vi "Weather Parse Test.vi"() -> ()   [LabVIEW 2020, in "CDM-Config.lvlib"] (continued)
 \"SMALL CRAFT ADVISORY THROUGH WEDNESDAY NIGHT\"\n                    ],\n                    \"BLOCKCHANNEL\": [\n                        \"EAS\",\n                        \"NWEM\",\n                        \"CMAS\"\n                    ],\n                    \"VTEC\": [\n                        \"/O.NEW.PAFC.SC.Y.7456.251203T1400Z-251204T1400Z/\"\n                    ],\n                    \"eventEndingTime\": [\n                        \"2025-12-04T05:00:00-09:00\"\n                    ]\n                },\n                \"scope\": \"Public\",\n                \"code\": \"IPAWSv1.0\",\n                \"language\": \"en-US\",\n                \"web\": \"http://www.weather.gov\",\n                \"eventCode\": {\n                    \"SAME\": [\n                        \"NWS\"\n                    ],\n                    \"NationalWeatherService\": [\n                        \"SCY\"\n                    ]\n                }\n            }\n        },\n        {\n            \"id\": \"https://api.weather.gov/alerts/urn:oid:2.49.0.1.840.0.1f582400c49c338dd966fa4e73bebf0ceb9d5ea9.006.1\",\n            \"type\": \"Feature\",\n            \"geometry\": null,\n            \"properties\": {\n                \"@id\": \"https://api.weather.gov/alerts/urn:oid:2.49.0.1.840.0.1f582400c49c338dd966fa4e73bebf0ceb9d5ea9.006.1\",\n                \"@type\": \"wx:Alert\",\n                \"id\": \"urn:oid:2.49.0.1.840.0.1f582400c49c338dd966fa4e73bebf0ceb9d5ea9.006.1\",\n                \"areaDesc\": \"Cape Cleare to Gore Point from 15 to 75 NM\",\n                \"geocode\": {\n                    \"SAME\": [\n                        \"058716\"\n                    ],\n                    \"UGC\": [\n                        \"PKZ716\"\n                    ]\n                },\n                \"affectedZones\": [\n                    \"https://api.weather.gov/zones/forecast/PKZ716\"\n                ],\n                \"references\": [],\n                \"sent\": \"2025-12-02T15:47:00-09:00\",\n                \"effective\": \"2025-12-02T15:47:00-09:00\",\n                \"onset\": \"2025-12-03T05:00:00-09:00\",\n                \"expires\": \"2025-12-03T04:45:00-09:00\",\n                \"ends\": \"2025-12-04T05:00:00-09:00\",\n                \"status\": \"Actual\",\n                \"messageType\": \"Alert\",\n                \"category\": \"Met\",\n                \"severity\": \"Minor\",\n                \"certainty\": \"Likely\",\n                \"urgency\": \"Expected\",\n                \"event\": \"Small Craft Advisory\",\n                \"sender\": \"w-nws.webmaster@noaa.gov\",\n                \"senderName\": \"NWS Anchorage AK\",\n                \"headline\": \"Small Craft Advisory issued December 2 at 3:47PM AKST until December 4 at 5:00AM AKST by NWS Anchorage AK\",\n                \"description\": \"Coastal Waters Forecast for the Northern Gulf of Alaska Coast\\nup to 100 nm out including Kodiak Island and Cook Inlet.\\n\\nWind forecasts reflect the predominant speed and direction\\nexpected. Sea forecasts represent an average of the highest\\none-third of the combined wind wave and swell height.\\n\\n.TONIGHT...Variable wind 10 kt. Seas 11 ft.\\n.WED...Variable wind 10 kt. Seas 10 ft.\\n.WED NIGHT...SW wind 15 kt. Seas 10 ft.\\n.THU AND THU NIGHT...Variable wind 10 kt. Seas 8 ft.\\n.FRI...NW wind 20 kt. Seas 6 ft.\\n.SAT...SE wind 15 kt. Seas 7 ft.\\n.SUN...E wind 15 kt. Seas 11 ft.\",\n                \"instruction\": null,\n                \"response\": \"Avoid\",\n                \"parameters\": {\n                    \"AWIPSidentifier\": [\n                        \"CWFAER\"\n                    ],\n                    \"WMOidentifier\": [\n                        \"FZAK51 PAFC 030047\"\n                    ],\n                    \"NWSheadline\": [\n                        \"SMALL CRAFT ADVISORY THROUGH WEDNESDAY NIGHT\"\n                    ],\n                    \"BLOCKCHANNEL\": [\n                        \"EAS\",\n                        \"NWEM\",\n                        \"CMAS\"\n                    ],\n                    \"VTEC\": [\n                        \"/O.NEW.PAFC.SC.Y.7452.251203T1400Z-251204T1400Z/\"\n                    ],\n                    \"eventEndingTime\": [\n                        \"2025-12-04T05:00:00-09:00\"\n                    ]\n                },\n                \"scope\": \"Public\",\n                \"code\": \"IPAWSv1.0\",\n                \"language\": \"en-US\",\n                \"web\": \"http://www.weather.gov\",\n                \"eventCode\": {\n                    \"SAME\": [\n                        \"NWS\"\n                    ],\n                    \"NationalWeatherService\": [\n                        \"SCY\"\n                    ]\n                }\n            }\n        },\n        {\n            \"id\": \"https://api.weather.gov/alerts/urn:oid:2.49.0.1.840.0.1f582400c49c338dd966fa4e73bebf0ceb9d5ea9.017.1\",\n            \"type\": \"Feature\",\n            \"geometry\": null,\n            \"properties\": {\n                \"@id\": \"https://api.weather.gov/alerts/urn:oid:2.49.0.1.840.0.1f582400c49c338dd966fa4e73bebf0ceb9d5ea9.017.1\",\n                \"@type\": \"wx:Alert\",\n                \"id\": \"urn:oid:2.49.0.1.840.0.1f582400c49c338dd966fa4e73bebf0ceb9d5ea9.017.1\",\n                \"areaDesc\": \"Gore Point to Marmot Island from 15 to 80 NM\",\n                \"geocode\": {\n                    \"SAME\": [\n                        \"058733\"\n                    ],\n                    \"UGC\": [\n                        \"PKZ733\"\n                    ]\n                },\n                \"affectedZones\": [\n                    \"https://api.weather.gov/zones/forecast/PKZ733\"\n                ],\n                \"references\": [],\n                \"sent\": \"2025-12-02T15:47:00-09:00\",\n                \"effective\": \"2025-12-02T15:47:00-09:00\",\n                \"onset\": \"2025-12-03T05:00:00-09:00\",\n                \"expires\": \"2025-12-03T04:45:00-09:00\",\n                \"ends\": \"2025-12-04T05:00:00-09:00\",\n                \"status\": \"Actual\",\n                \"messageType\": \"Alert\",\n                \"category\": \"Met\",\n                \"severity\": \"Minor\",\n                \"certainty\": \"Likely\",\n                \"urgency\": \"Expected\",\n                \"event\": \"Small Craft Advisory\",\n                \"sender\": \"w-nws.webmaster@noaa.gov\",\n                \"senderName\": \"NWS Anchorage AK\",\n                \"headline\": \"Small Craft Advisory issued December 2 at 3:47PM AKST until December 4 at 5:00AM AKST by NWS Anchorage AK\",\n                \"description\": \"Coastal Waters Forecast for the Northern Gulf of Alaska Coast\\nup to 100 nm out including Kodiak Island and Cook Inlet.\\n\\nWind forecasts reflect the predominant speed and direction\\nexpected. Sea forecasts represent an average of the highest\\none-third of the combined wind wave and swell height.\\n\\n.TONIGHT...SE wind 15 kt. Seas 11 ft.\\n.WED...SE wind 15 kt. Seas 11 ft.\\n.WED NIGHT...SW wind 15 kt. Seas 9 ft.\\n.THU...SW wind 15 kt. Seas 8 ft.\\n.THU NIGHT...Variable wind 10 kt. Seas 7 ft.\\n.FRI...NW wind 15 kt. Seas 9 ft.\\n.SAT...Variable wind 10 kt. Seas 9 ft.\\n.SUN...E wind 15 kt. Seas 9 ft.\",\n                \"instruction\": null,\n                \"response\": \"Avoid\",\n                \"parameters\": {\n                    \"AWIPSidentifier\": [\n                        \"CWFAER\"\n                    ],\n                    \"WMOidentifier\": [\n                        \"FZAK51 PAFC 030047\"\n                    ],\n                    \"NWSheadline\": [\n                        \"SMALL CRAFT ADVISORY THROUGH WEDNESDAY NIGHT\"\n                    ],\n                    \"BLOCKCHANNEL\": [\n                        \"EAS\",\n                        \"NWEM\",\n                        \"CMAS\"\n                    ],\n                    \"VTEC\": [\n                        \"/O.NEW.PAFC.SC.Y.7454.251203T1400Z-251204T1400Z/\"\n                    ],\n                    \"eventEndingTime\": [\n                        \"2025-12-04T05:00:00-09:00\"\n                    ]\n                },\n                \"scope\": \"Public\",\n                \"code\": \"IPAWSv1.0\",\n                \"language\": \"en-US\",\n                \"web\": \"http://www.weather.gov\",\n                \"eventCode\": {\n                    \"SAME\": [\n                        \"NWS\"\n                    ],\n                    \"NationalWeatherService\": [\n                        \"SCY\"\n                    ]\n                }\n            }\n        },\n        {\n            \"id\": \"https://api.weather.gov/alerts/urn:oid:2.49.0.1.840.0.1f582400c49c338dd966fa4e73bebf0ceb9d5ea9.003.1\",\n            \"type\": \"Feature\",\n            \"geometry\": null,\n            \"properties\": {\n                \"@id\": \"https://api.weather.gov/alerts/urn:oid:2.49.0.1.840.0.1f582400c49c338dd966fa4e73bebf0ceb9d5ea9.003.1\",\n                \"@type\": \"wx:Alert\",\n                \"id\": \"urn:oid:2.49.0.1.840.0.1f582400c49c338dd966fa4e73bebf0ceb9d5ea9.003.1\",\n                \"areaDesc\": \"Gravel Point to Cape Cleare out to 15 NM\",\n                \"geocode\": {\n                    \"SAME\": [\n                        \"058711\"\n                    ],\n                    \"UGC\": [\n                        \"PKZ711\"\n                    ]\n                },\n                \"affectedZones\": [\n                    \"https://api.weather.gov/zones/forecast/PKZ711\"\n                ],\n                \"references\": [],\n                \"sent\": \"2025-12-02T15:47:00-09:00\",\n                \"effective\": \"2025-12-02T15:47:00-09:00\",\n                \"onset\": \"2025-12-03T05:00:00-09:00\",\n                \"expires\": \"2025-12-03T04:45:00-09:00\",\n                \"ends\": \"2025-12-04T05:00:00-09:00\",\n                \"status\": \"Actual\",\n                \"messageType\": \"Alert\",\n                \"category\": \"Met\",\n                \"severity\": \"Minor\",\n                \"certainty\": \"Likely\",\n                \"urgency\": \"Expected\",\n                \"event\": \"Small Craft Advisory\",\n                \"sender\": \"w-nws.webmaster@noaa.gov\",\n                \"senderName\": \"NWS Anchorage AK\",\n                \"headline\": \"Small Craft Advisory issued December 2 at 3:47PM AKST until December 4 at 5:00AM AKST by NWS Anchorage AK\",\n                \"description\": \"Coastal Waters Forecast for the Northern Gulf of Alaska Coast\\nup to 100 nm out including Kodiak Island and Cook Inlet.\\n\\nWind forecasts reflect the predominant speed and direction\\nexpected. Sea forecasts represent an average of the highest\\none-third of the combined wind wave and swell height.\\n\\n.TONIGHT...SE wind 25 kt. Seas 10 ft.\\n.WED...SE wind 15 kt in the morning becoming variable 10 kt. Seas\\n10 ft. Rain.\\n.WED NIGHT...Variable wind 10 kt. Seas 9 ft.\\n.THU...Variable wind 10 kt. Seas 7 ft.\\n.THU NIGHT...Variable wind 10 kt. Seas 6 ft.\\n.FRI...NE wind 15 kt. Seas 6 ft.\\n.SAT THROUGH SUN...E wind 20 kt. Seas 10 ft.\",\n                \"instruction\": null,\n                \"response\": \"Avoid\",\n                \"parameters\": {\n                    \"AWIPSidentifier\": [\n                        \"CWFAER\"\n                    ],\n                    \"WMOidentifier\": [\n                        \"FZAK51 PAFC 030047\"\n                    ],\n                    \"NWSheadline\": [\n                        \"SMALL CRAFT ADVISORY THROUGH WEDNESDAY NIGHT\"\n                    ],\n                    \"BLOCKCHANNEL\": [\n                        \"EAS\",\n                        \"NWEM\",\n                        \"CMAS\"\n                    ],\n                    \"VTEC\": [\n                        \"/O.NEW.PAFC.SC.Y.7449.251203T1400Z-251204T1400Z/\"\n                    ],\n                    \"eventEndingTime\": [\n                        \"2025-12-04T05:00:00-09:00\"\n                    ]\n                },\n                \"scope\": \"Public\",\n                \"code\": \"IPAWSv1.0\",\n                \"language\": \"en-US\",\n                \"web\": \"http://www.weather.gov\",\n                \"eventCode\": {\n                    \"SAME\": [\n                        \"NWS\"\n                    ],\n                    \"NationalWeatherService\": [\n                        \"SCY\"\n                    ]\n                }\n            }\n        },\n        {\n            \"id\": \"https://api.weather.gov/alerts/urn:oid:2.49.0.1.840.0.1f582400c49c338dd966fa4e73bebf0ceb9d5ea9.018.1\",\n            \"type\": \"Feature\",\n            \"geometry\": null,\n            \"properties\": {\n                \"@id\": \"https://api.weather.gov/alerts/urn:oid:2.49.0.1.840.0.1f582400c49c338dd966fa4e73bebf0ceb9d5ea9.018.1\",\n                \"@type\": \"wx:Alert\",\n                \"id\": \"urn:oid:2.49.0.1.840.0.1f582400c49c338dd966fa4e73bebf0ceb9d5ea9.018.1\",\n                \"areaDesc\": \"Marmot Island to Sitkinak out to 15 NM\",\n                \"geocode\": {\n                    \"SAME\": [\n                        \"058732\"\n                    ],\n                    \"UGC\": [\n                        \"PKZ732\"\n                    ]\n                },\n                \"affectedZones\": [\n                    \"https://api.weather.gov/zones/forecast/PKZ732\"\n                ],\n                \"references\": [],\n                \"sent\": \"2025-12-02T15:47:00-09:00\",\n                \"effective\": \"2025-12-02T15:47:00-09:00\",\n                \"onset\": \"2025-12-03T05:00:00-09:00\",\n                \"expires\": \"2025-12-03T04:45:00-09:00\",\n                \"ends\": \"2025-12-04T05:00:00-09:00\",\n                \"status\": \"Actual\",\n                \"messageType\": \"Alert\",\n                \"category\": \"Met\",\n                \"severity\": \"Minor\",\n                \"certainty\": \"Likely\",\n                \"urgency\": \"Expected\",\n                \"event\": \"Small Craft Advisory\",\n                \"sender\": \"w-nws.webmaster@noaa.gov\",\n                \"senderName\": \"NWS Anchorage AK\",\n                \"headline\": \"Small Craft Advisory issued December 2 at 3:47PM AKST until December 4 at 5:00AM AKST by NWS Anchorage AK\",\n                \"description\": \"Coastal Waters Forecast for the Northern Gulf of Alaska Coast\\nup to 100 nm out including Kodiak Island and Cook Inlet.\\n\\nWind forecasts reflect the predominant speed and direction\\nexpected. Sea forecasts represent an average of the highest\\none-third of the combined wind wave and swell height.\\n\\n.TONIGHT...E wind 20 kt. Seas 13 ft.\\n.WED...S wind 20 kt. Seas 12 ft.\\n.WED NIGHT...S wind 15 kt. Seas 9 ft.\\n.THU...SE wind 15 kt. Seas 9 ft.\\n.THU NIGHT...NE wind 20 kt. Seas 9 ft.\\n.FRI THROUGH SUN...W wind 20 kt. Seas 7 ft.\",\n                \"instruction\": null,\n                \"response\": \"Avoid\",\n                \"parameters\": {\n                    \"AWIPSidentifier\": [\n                        \"CWFAER\"\n                    ],\n                    \"WMOidentifier\": [\n                        \"FZAK51 PAFC 030047\"\n                    ],\n                    \"NWSheadline\": [\n                        \"SMALL CRAFT ADVISORY THROUGH WEDNESDAY NIGHT\"\n                    ],\n                    \"BLOCKCHANNEL\": [\n                        \"EAS\",\n                        \"NWEM\",\n                        \"CMAS\"\n                    ],\n                    \"VTEC\": [\n                        \"/O.NEW.PAFC.SC.Y.7455.251203T1400Z-251204T1400Z/\"\n                    ],\n                    \"eventEndingTime\": [\n                        \"2025-12-04T05:00:00-09:00\"\n                    ]\n                },\n                \"scope\": \"Public\",\n                \"code\": \"IPAWSv1.0\",\n                \"language\": \"en-US\",\n                \"web\": \"http://www.weather.gov\",\n                \"eventCode\": {\n                    \"SAME\": [\n                        \"NWS\"\n                    ],\n                    \"NationalWeatherService\": [\n                        \"SCY\"\n                    ]\n                }\n            }\n        },\n        {\n            \"id\": \"https://api.weather.gov/alerts/urn:oid:2.49.0.1.840.0.1f582400c49c338dd966fa4e73bebf0ceb9d5ea9.004.1\",\n            \"type\": \"Feature\",\n            \"geometry\": null,\n            \"properties\": {\n                \"@id\": \"https://api.weather.gov/alerts/urn:oid:2.49.0.1.840.0.1f582400c49c338dd966fa4e73bebf0ceb9d5ea9.004.1\",\n                \"@type\": \"wx:Alert\",\n                \"id\": \"urn:oid:2.49.0.1.840.0.1f582400c49c338dd966fa4e73bebf0ceb9d5ea9.004.1\",\n                \"areaDesc\": \"Cape Suckling to Cape Cleare from 15 to 75 NM\",\n                \"geocode\": {\n                    \"SAME\": [\n                        \"058712\"\n                    ],\n                    \"UGC\": [\n                        \"PKZ712\"\n                    ]\n                },\n                \"affectedZones\": [\n                    \"https://api.weather.gov/zones/forecast/PKZ712\"\n                ],\n                \"references\": [],\n                \"sent\": \"2025-12-02T15:47:00-09:00\",\n                \"effective\": \"2025-12-02T15:47:00-09:00\",\n                \"onset\": \"2025-12-03T05:00:00-09:00\",\n                \"expires\": \"2025-12-03T04:45:00-09:00\",\n                \"ends\": \"2025-12-04T05:00:00-09:00\",\n                \"status\": \"Actual\",\n                \"messageType\": \"Alert\",\n                \"category\": \"Met\",\n                \"severity\": \"Minor\",\n                \"certainty\": \"Likely\",\n                \"urgency\": \"Expected\",\n                \"event\": \"Small Craft Advisory\",\n                \"sender\": \"w-nws.webmaster@noaa.gov\",\n                \"senderName\": \"NWS Anchorage AK\",\n                \"headline\": \"Small Craft Advisory issued December 2 at 3:47PM AKST until December 4 at 5:00AM AKST by NWS Anchorage AK\",\n                \"description\": \"Coastal Waters Forecast for the Northern Gulf of Alaska Coast\\nup to 100 nm out including Kodiak Island and Cook Inlet.\\n\\nWind forecasts reflect the predominant speed and direction\\nexpected. Sea forecasts represent an average of the highest\\none-third of the combined wind wave and swell height.\\n\\n.TONIGHT...SE wind 25 kt. Seas 10 ft.\\n.WED...S wind 15 kt. Seas 11 ft.\\n.WED NIGHT...SW wind 15 kt. Seas 10 ft.\\n.THU...SW wind 15 kt. Seas 8 ft.\\n.THU NIGHT...Variable wind 10 kt. Seas 8 ft.\\n.FRI...S wind 15 kt. Seas 7 ft.\\n.SAT THROUGH SUN...SE wind 20 kt. Seas 11 ft.\",\n                \"instruction\": null,\n                \"response\": \"Avoid\",\n                \"parameters\": {\n                    \"AWIPSidentifier\": [\n                        \"CWFAER\"\n                    ],\n                    \"WMOidentifier\": [\n                        \"FZAK51 PAFC 030047\"\n                    ],\n                    \"NWSheadline\": [\n                        \"SMALL CRAFT ADVISORY THROUGH WEDNESDAY NIGHT\"\n                    ],\n                    \"BLOCKCHANNEL\": [\n                        \"EAS\",\n                        \"NWEM\",\n                        \"CMAS\"\n                    ],\n                    \"VTEC\": [\n                        \"/O.NEW.PAFC.SC.Y.7450.251203T1400Z-251204T1400Z/\"\n                    ],\n                    \"eventEndingTime\": [\n                        \"2025-12-04T05:00:00-09:00\"\n                    ]\n                },\n                \"scope\": \"Public\",\n                \"code\": \"IPAWSv1.0\",\n                \"language\": \"en-US\",\n                \"web\": \"http://www.weather.gov\",\n                \"eventCode\": {\n                    \"SAME\": [\n                        \"NWS\"\n                    ],\n                    \"NationalWeatherService\": [\n                        \"SCY\"\n                    ]\n                }\n            }\n        },\n        {\n            \"id\": \"https://api.weather.gov/alerts/urn:oid:2.49.0.1.840.0.ddc072ff7c65d7dc76b55ecdda687f2ed71d6895.001.1\",\n            \"type\": \"Feature\",\n            \"geometry\": null,\n            \"properties\": {\n                \"@id\": \"https://api.weather.gov/alerts/urn:oid:2.49.0.1.840.0.ddc072ff7c65d7dc76b55ecdda687f2ed71d6895.001.1\",\n                \"@type\": \"wx:Alert\",\n                \"id\": \"urn:oid:2.49.0.1.840.0.ddc072ff7c65d7dc76b55ecdda687f2ed71d6895.001.1\",\n                \"areaDesc\": \"Yakutat Bay\",\n                \"geocode\": {\n                    \"SAME\": [\n                        \"058053\"\n                    ],\n                    \"UGC\": [\n                        \"PKZ053\"\n                    ]\n                },\n                \"affectedZones\": [\n                    \"https://api.weather.gov/zones/forecast/PKZ053\"\n                ],\n                \"references\": [],\n                \"sent\": \"2025-12-02T14:58:00-09:00\",\n                \"effective\": \"2025-12-02T14:58:00-09:00\",\n                \"onset\": \"2025-12-02T14:00:00-09:00\",\n                \"expires\": \"2025-12-03T09:00:00-09:00\",\n                \"ends\": \"2025-12-03T17:00:00-09:00\",\n                \"status\": \"Actual\",\n                \"messageType\": \"Alert\",\n                \"category\": \"Met\",\n                \"severity\": \"Minor\",\n                \"certainty\": \"Likely\",\n                \"urgency\": \"Expected\",\n                \"event\": \"Small Craft Advisory\",\n                \"sender\": \"w-nws.webmaster@noaa.gov\",\n                \"senderName\": \"NWS Juneau AK\",\n                \"headline\": \"Small Craft Advisory issued December 2 at 2:58PM AKST until December 3 at 5:00PM AKST by NWS Juneau AK\",\n                \"description\": \"Coastal Waters Forecast for Yakutat Bay\\n\\nWind forecasts reflect the predominant speed and direction\\nexpected. Sea forecasts represent the average of the highest\\none-third of the combined windwave and swell height.\\n\\n.TONIGHT...E wind 15 kt. Seas 9 ft. Rain.\\n.WED...E wind 15 kt. Seas 10 ft. S swell. Rain.\\n.WED NIGHT...S wind 10 kt in the evening becoming light.\\nSeas 9 ft. S swell. Rain.\\n.THU...E wind 10 kt. Seas 8 ft. SW swell. Rain.\\n.THU NIGHT...E wind 15 kt. Seas 7 ft. SW swell. Rain.\\n.FRI...E wind 25 kt. Seas 7 ft.\\n.SAT...E gale to 35 kt. Seas 10 ft.\\n.SUN...E gale to 35 kt. Seas 12 ft.\",\n                \"instruction\": null,\n                \"response\": \"Avoid\",\n                \"parameters\": {\n                    \"AWIPSidentifier\": [\n                        \"CWFYAK\"\n                    ],\n                    \"WMOidentifier\": [\n                        \"FZAK53 PAJK 022358\"\n                    ],\n                    \"NWSheadline\": [\n                        \"SMALL CRAFT ADVISORY THROUGH WEDNESDAY\"\n                    ],\n                    \"BLOCKCHANNEL\": [\n                        \"EAS\",\n                        \"NWEM\",\n                        \"CMAS\"\n                    ],\n                    \"VTEC\": [\n                        \"/O.NEW.PAJK.SC.Y.5129.251202T2300Z-251204T0200Z/\"\n                    ],\n                    \"eventEndingTime\": [\n                        \"2025-12-03T17:00:00-09:00\"\n                    ]\n                },\n                \"scope\": \"Public\",\n                \"code\": \"IPAWSv1.0\",\n                \"language\": \"en-US\",\n                \"web\": \"http://www.weather.gov\",\n                \"eventCode\": {\n                    \"SAME\": [\n                        \"NWS\"\n                    ],\n                    \"NationalWeatherService\": [\n                        \"SCY\"\n                    ]\n                }\n            }\n        },\n        {\n            \"id\": \"https://api.weather.gov/alerts/urn:oid:2.49.0.1.840.0.cf65336ecbc386541a5c0d1a125271af790bff70.006.1\",\n            \"type\": \"Feature\",\n            \"geometry\": null,\n            \"properties\": {\n                \"@id\": \"https://api.weather.gov/alerts/urn:oid:2.49.0.1.840.0.cf65336ecbc386541a5c0d1a125271af790bff70.006.1\",\n                \"@type\": \"wx:Alert\",\n                \"id\": \"urn:oid:2.49.0.1.840.0.cf65336ecbc386541a5c0d1a125271af790bff70.006.1\",\n                \"areaDesc\": \"Cross Sound\",\n                \"geocode\": {\n                    \"SAME\": [\n                        \"058022\"\n                    ],\n                    \"UGC\": [\n                        \"PKZ022\"\n                    ]\n                },\n                \"affectedZones\": [\n                    \"https://api.weather.gov/zones/forecast/PKZ022\"\n                ],\n                \"references\": [],\n                \"sent\": \"2025-12-02T14:58:00-09:00\",\n                \"effective\": \"2025-12-02T14:58:00-09:00\",\n                \"onset\": \"2025-12-02T14:00:00-09:00\",\n                \"expires\": \"2025-12-03T07:30:00-09:00\",\n                \"ends\": \"2025-12-03T17:00:00-09:00\",\n                \"status\": \"Actual\",\n                \"messageType\": \"Alert\",\n                \"category\": \"Met\",\n                \"severity\": \"Minor\",\n                \"certainty\": \"Likely\",\n                \"urgency\": \"Expected\",\n                \"event\": \"Small Craft Advisory\",\n                \"sender\": \"w-nws.webmaster@noaa.gov\",\n                \"senderName\": \"NWS Juneau AK\",\n                \"headline\": \"Small Craft Advisory issued December 2 at 2:58PM AKST until December 3 at 5:00PM AKST by NWS Juneau AK\",\n                \"description\": \"Southeast Alaska Inside Waters from Dixon Entrance to Skagway\\n\\nWind forecasts reflect the predominant speed and direction\\nexpected. Sea forecasts represent the average of the highest\\none-third of the combined windwave and swell height.\\n\\n.TONIGHT...S wind 15 kt becoming E. Seas 9 ft. Rain.\\n.WED...NE wind 15 kt becoming SW in the afternoon. Seas\\n9 ft. S swell. Rain.\\n.WED NIGHT...W wind 15 kt. Seas 8 ft. S swell. Rain.\\n.THU...W wind 15 kt. Seas 8 ft. Rain.\\n.THU NIGHT...NE wind 10 kt. Seas 7 ft. Rain.\\n.FRI...NE wind 15 kt. Seas 7 ft.\\n.SAT...S wind 25 kt. Seas 8 ft.\\n.SUN...SE wind 30 kt. Seas 11 ft.\",\n                \"instruction\": null,\n                \"response\": \"Avoid\",\n                \"parameters\": {\n                    \"AWIPSidentifier\": [\n                        \"CWFAJK\"\n                    ],\n                    \"WMOidentifier\": [\n                        \"FZAK51 PAJK 022358\"\n                    ],\n                    \"NWSheadline\": [\n                        \"SMALL CRAFT ADVISORY THROUGH WEDNESDAY\"\n                    ],\n                    \"BLOCKCHANNEL\": [\n                        \"EAS\",\n                        \"NWEM\",\n                        \"CMAS\"\n                    ],\n                    \"VTEC\": [\n                        \"/O.NEW.PAJK.SC.Y.2507.251202T2300Z-251204T0200Z/\"\n                    ],\n                    \"eventEndingTime\": [\n                        \"2025-12-03T17:00:00-09:00\"\n                    ]\n                },\n                \"scope\": \"Public\",\n                \"code\": \"IPAWSv1.0\",\n                \"language\": \"en-US\",\n                \"web\": \"http://www.weather.gov\",\n                \"eventCode\": {\n                    \"SAME\": [\n                        \"NWS\"\n                    ],\n                    \"NationalWeatherService\": [\n                        \"SCY\"\n                    ]\n                }\n            }\n        },\n        {\n            \"id\": \"https://api.weather.gov/alerts/urn:oid:2.49.0.1.840.0.cf65336ecbc386541a5c0d1a125271af790bff70.012.1\",\n            \"type\": \"Feature\",\n            \"geometry\": null,\n            \"properties\": {\n                \"@id\": \"https://api.weather.gov/alerts/urn:oid:2.49.0.1.840.0.cf65336ecbc386541a5c0d1a125271af790bff70.012.1\",\n                \"@type\": \"wx:Alert\",\n                \"id\": \"urn:oid:2.49.0.1.840.0.cf65336ecbc386541a5c0d1a125271af790bff70.012.1\",\n                \"areaDesc\": \"Clarence Strait\",\n                \"geocode\": {\n                    \"SAME\": [\n                        \"058036\"\n                    ],\n                    \"UGC\": [\n                        \"PKZ036\"\n                    ]\n                },\n                \"affectedZones\": [\n                    \"https://api.weather.gov/zones/forecast/PKZ036\"\n                ],\n                \"references\": [],\n                \"sent\": \"2025-12-02T14:58:00-09:00\",\n                \"effective\": \"2025-12-02T14:58:00-09:00\",\n                \"onset\": \"2025-12-02T17:00:00-09:00\",\n                \"expires\": \"2025-12-03T07:30:00-09:00\",\n                \"ends\": \"2025-12-03T17:00:00-09:00\",\n                \"status\": \"Actual\",\n                \"messageType\": \"Alert\",\n                \"category\": \"Met\",\n                \"severity\": \"Minor\",\n                \"certainty\": \"Likely\",\n                \"urgency\": \"Expected\",\n                \"event\": \"Small Craft Advisory\",\n                \"sender\": \"w-nws.webmaster@noaa.gov\",\n                \"senderName\": \"NWS Juneau AK\",\n                \"headline\": \"Small Craft Advisory issued December 2 at 2:58PM AKST until December 3 at 5:00PM AKST by NWS Juneau AK\",\n                \"description\": \"Southeast Alaska Inside Waters from Dixon Entrance to Skagway\\n\\nWind forecasts reflect the predominant speed and direction\\nexpected. Sea forecasts represent the average of the highest\\none-third of the combined windwave and swell height.\\n\\n.TONIGHT...S wind 15 kt becoming SE 25 kt late. Seas building to\\n4 ft. Near ocean entrances, seas 7 ft. Rain.\\n.WED...S wind 20 kt. Seas 8 ft, except 11 ft near ocean\\nentrances. Rain.\\n.WED NIGHT...SW wind 10 kt. Seas 4 ft, except 7 ft near\\nocean entrances.\\n.THU...S wind 10 kt. Seas 3 ft.\\n.THU NIGHT...E wind 20 kt. Seas 5 ft. Rain.\\n.FRI...S wind 20 kt. Seas 6 ft.\\n.SAT...S gale to 40 kt. Seas 12 ft.\\n.SUN...S gale to 45 kt. Seas 14 ft.\",\n                \"instruction\": null,\n                \"response\": \"Avoid\",\n                \"parameters\": {\n                    \"AWIPSidentifier\": [\n                        \"CWFAJK\"\n                    ],\n                    \"WMOidentifier\": [\n                        \"FZAK51 PAJK 022358\"\n                    ],\n                    \"NWSheadline\": [\n                        \"SMALL CRAFT ADVISORY LATE TONIGHT THROUGH WEDNESDAY\"\n                    ],\n                    \"BLOCKCHANNEL\": [\n                        \"EAS\",\n                        \"NWEM\",\n                        \"CMAS\"\n                    ],\n                    \"VTEC\": [\n                        \"/O.NEW.PAJK.SC.Y.2510.251203T0200Z-251204T0200Z/\"\n                    ],\n                    \"eventEndingTime\": [\n                        \"2025-12-03T17:00:00-09:00\"\n                    ]\n                },\n                \"scope\": \"Public\",\n                \"code\": \"IPAWSv1.0\",\n                \"language\": \"en-US\",\n                \"web\": \"http://www.weather.gov\",\n                \"eventCode\": {\n                    \"SAME\": [\n                        \"NWS\"\n                    ],\n                    \"NationalWeatherService\": [\n                        \"SCY\"\n                    ]\n                }\n            }\n        },\n        {\n            \"id\": \"https://api.weather.gov/alerts/urn:oid:2.49.0.1.840.0.cf65336ecbc386541a5c0d1a125271af790bff70.010.1\",\n            \"type\": \"Feature\",\n            \"geometry\": null,\n            \"properties\": {\n                \"@id\": \"https://api.weather.gov/alerts/urn:oid:2.49.0.1.840.0.cf65336ecbc386541a5c0d1a125271af790bff70.010.1\",\n                \"@type\": \"wx:Alert\",\n                \"id\": \"urn:oid:2.49.0.1.840.0.cf65336ecbc386541a5c0d1a125271af790bff70.010.1\",\n                \"areaDesc\": \"Frederick Sound\",\n                \"geocode\": {\n                    \"SAME\": [\n                        \"058034\"\n                    ],\n                    \"UGC\": [\n                        \"PKZ034\"\n                    ]\n                },\n                \"affectedZones\": [\n                    \"https://api.weather.gov/zones/forecast/PKZ034\"\n                ],\n                \"references\": [],\n                \"sent\": \"2025-12-02T14:58:00-09:00\",\n                \"effective\": \"2025-12-02T14:58:00-09:00\",\n                \"onset\": \"2025-12-02T17:00:00-09:00\",\n                \"expires\": \"2025-12-03T07:30:00-09:00\",\n                \"ends\": \"2025-12-03T17:00:00-09:00\",\n                \"status\": \"Actual\",\n                \"messageType\": \"Alert\",\n                \"category\": \"Met\",\n                \"severity\": \"Minor\",\n                \"certainty\": \"Likely\",\n                \"urgency\": \"Expected\",\n                \"event\": \"Small Craft Advisory\",\n                \"sender\": \"w-nws.webmaster@noaa.gov\",\n                \"senderName\": \"NWS Juneau AK\",\n                \"headline\": \"Small Craft Advisory issued December 2 at 2:58PM AKST until December 3 at 5:00PM AKST by NWS Juneau AK\",\n                \"description\": \"Southeast Alaska Inside Waters from Dixon Entrance to Skagway\\n\\nWind forecasts reflect the predominant speed and direction\\nexpected. Sea forecasts represent the average of the highest\\none-third of the combined windwave and swell height.\\n\\n.TONIGHT...SE wind 15 kt becoming 25 kt late. Seas 4 ft. Patchy\\nfog in the evening. Rain.\\n.WED...SE wind 25 kt diminishing to 15 kt in the afternoon.\\nSeas 4 ft. Rain.\\n.WED NIGHT...S wind 15 kt. Seas 3 ft in the evening then\\n2 ft or less.\\n.THU...S wind 10 kt. Seas 2 ft or less.\\n.THU NIGHT...E wind 10 kt. Seas 2 ft or less. Rain.\\n.FRI...SE wind 20 kt. Seas 4 ft.\\n.SAT...SE wind 30 kt. Seas 6 ft.\\n.SUN...SE gale to 35 kt. Seas 7 ft.\",\n                \"instruction\": null,\n                \"response\": \"Avoid\",\n                \"parameters\": {\n                    \"AWIPSidentifier\": [\n                        \"CWFAJK\"\n                    ],\n                    \"WMOidentifier\": [\n                        \"FZAK51 PAJK 022358\"\n                    ],\n                    \"NWSheadline\": [\n                        \"SMALL CRAFT ADVISORY LATE TONIGHT THROUGH WEDNESDAY\"\n                    ],\n                    \"BLOCKCHANNEL\": [\n                        \"EAS\",\n                        \"NWEM\",\n                        \"CMAS\"\n                    ],\n                    \"VTEC\": [\n                        \"/O.NEW.PAJK.SC.Y.2509.251203T0200Z-251204T0200Z/\"\n                    ],\n                    \"eventEndingTime\": [\n                        \"2025-12-03T17:00:00-09:00\"\n                    ]\n                },\n                \"scope\": \"Public\",\n                \"code\": \"IPAWSv1.0\",\n                \"language\": \"en-US\",\n                \"web\": \"http://www.weather.gov\",\n                \"eventCode\": {\n                    \"SAME\": [\n                        \"NWS\"\n                    ],\n                    \"NationalWeatherService\": [\n                        \"SCY\"\n                    ]\n                }\n            }\n        },\n        {\n            \"id\": \"https://api.weather.gov/alerts/urn:oid:2.49.0.1.840.0.63d5e98d8e0beb997c67cb867ab3ed73fdae0812.003.1\",\n            \"type\": \"Feature\",\n            \"geometry\": null,\n            \"properties\": {\n                \"@id\": \"https://api.weather.gov/alerts/urn:oid:2.49.0.1.840.0.63d5e98d8e0beb997c67cb867ab3ed73fdae0812.003.1\",\n                \"@type\": \"wx:Alert\",\n                \"id\": \"urn:oid:2.49.0.1.840.0.63d5e98d8e0beb997c67cb867ab3ed73fdae0812.003.1\",\n                \"areaDesc\": \"Dixon Entrance to Cape Decision from 15 to 90 NM\",\n                \"geocode\": {\n                    \"SAME\": [\n                        \"058661\"\n                    ],\n                    \"UGC\": [\n                        \"PKZ661\"\n                    ]\n                },\n                \"affectedZones\": [\n                    \"https://api.weather.gov/zones/forecast/PKZ661\"\n                ],\n                \"references\": [],\n                \"sent\": \"2025-12-02T14:58:00-09:00\",\n                \"effective\": \"2025-12-02T14:58:00-09:00\",\n                \"onset\": \"2025-12-02T14:00:00-09:00\",\n                \"expires\": \"2025-12-03T09:00:00-09:00\",\n                \"ends\": \"2025-12-03T17:00:00-09:00\",\n                \"status\": \"Actual\",\n                \"messageType\": \"Alert\",\n                \"category\": \"Met\",\n                \"severity\": \"Minor\",\n                \"certainty\": \"Likely\",\n                \"urgency\": \"Expected\",\n                \"event\": \"Small Craft Advisory\",\n                \"sender\": \"w-nws.webmaster@noaa.gov\",\n                \"senderName\": \"NWS Juneau AK\",\n                \"headline\": \"Small Craft Advisory issued December 2 at 2:58PM AKST until December 3 at 5:00PM AKST by NWS Juneau AK\",\n                \"description\": \"Southeast Alaska Coastal Waters from Dixon Entrance to\\nCape Suckling out 100 NM\\n\\nWind forecasts reflect the predominant speed and direction\\nexpected. Seas forecasts represent the average of the highest\\none-third of the combined windwave and swell height.\\n\\n.TONIGHT...S wind 25 kt. Seas 11 ft. Rain.\\n.WED...W wind 15 kt. Seas 11 ft.\\n.WED NIGHT...W wind 15 kt. Seas 10 ft.\\n.THU...W wind 15 kt. Seas 8 ft. SW swell.\\n.THU NIGHT...SE wind 25 kt. Seas 9 ft. Rain.\\n.FRI...W wind 25 kt. Seas 17 ft.\\n.SAT...S gale to 35 kt. Seas 18 ft.\\n.SUN...SW gale to 35 kt. Seas 21 ft.\",\n                \"instruction\": null,\n                \"response\": \"Avoid\",\n                \"parameters\": {\n                    \"AWIPSidentifier\": [\n                        \"CWFAEG\"\n                    ],\n                    \"WMOidentifier\": [\n                        \"FZAK52 PAJK 022358\"\n                    ],\n                    \"NWSheadline\": [\n                        \"SMALL CRAFT ADVISORY THROUGH WEDNESDAY\"\n                    ],\n                    \"BLOCKCHANNEL\": [\n                        \"EAS\",\n                        \"NWEM\",\n                        \"CMAS\"\n                    ],\n                    \"VTEC\": [\n                        \"/O.NEW.PAJK.SC.Y.1224.251202T2300Z-251204T0200Z/\"\n                    ],\n                    \"eventEndingTime\": [\n                        \"2025-12-03T17:00:00-09:00\"\n                    ]\n                },\n                \"scope\": \"Public\",\n                \"code\": \"IPAWSv1.0\",\n                \"language\": \"en-US\",\n                \"web\": \"http://www.weather.gov\",\n                \"eventCode\": {\n                    \"SAME\": [\n                        \"NWS\"\n                    ],\n                    \"NationalWeatherService\": [\n                        \"SCY\"\n                    ]\n                }\n            }\n        },\n        {\n            \"id\": \"https://api.weather.gov/alerts/urn:oid:2.49.0.1.840.0.63d5e98d8e0beb997c67cb867ab3ed73fdae0812.008.1\",\n            \"type\": \"Feature\",\n            \"geometry\": null,\n            \"properties\": {\n                \"@id\": \"https://api.weather.gov/alerts/urn:oid:2.49.0.1.840.0.63d5e98d8e0beb997c67cb867ab3ed73fdae0812.008.1\",\n                \"@type\": \"wx:Alert\",\n                \"id\": \"urn:oid:2.49.0.1.840.0.63d5e98d8e0beb997c67cb867ab3ed73fdae0812.008.1\",\n                \"areaDesc\": \"Cape Spencer to Cape Fairweather out to 15 NM\",\n                \"geocode\": {\n                    \"SAME\": [\n                        \"058644\"\n                    ],\n                    \"UGC\": [\n                        \"PKZ644\"\n                    ]\n                },\n                \"affectedZones\": [\n                    \"https://api.weather.gov/zones/forecast/PKZ644\"\n                ],\n                \"references\": [],\n                \"sent\": \"2025-12-02T14:58:00-09:00\",\n                \"effective\": \"2025-12-02T14:58:00-09:00\",\n                \"onset\": \"2025-12-02T14:00:00-09:00\",\n                \"expires\": \"2025-12-03T09:00:00-09:00\",\n                \"ends\": \"2025-12-03T17:00:00-09:00\",\n                \"status\": \"Actual\",\n                \"messageType\": \"Alert\",\n                \"category\": \"Met\",\n                \"severity\": \"Minor\",\n                \"certainty\": \"Likely\",\n                \"urgency\": \"Expected\",\n                \"event\": \"Small Craft Advisory\",\n                \"sender\": \"w-nws.webmaster@noaa.gov\",\n                \"senderName\": \"NWS Juneau AK\",\n                \"headline\": \"Small Craft Advisory issued December 2 at 2:58PM AKST until December 3 at 5:00PM AKST by NWS Juneau AK\",\n                \"description\": \"Southeast Alaska Coastal Waters from Dixon Entrance to\\nCape Suckling out 100 NM\\n\\nWind forecasts reflect the predominant speed and direction\\nexpected. Seas forecasts represent the average of the highest\\none-third of the combined windwave and swell height.\\n\\n.TONIGHT...SE wind 15 kt increasing to 25 kt. Gusts to 40 kt.\\nSeas 11 ft. Rain.\\n.WED...E wind 25 kt becoming W 15 kt in the afternoon. Seas\\n12 ft. Rain.\\n.WED NIGHT...W wind 20 kt. Seas 10 ft.\\n.THU...W wind 15 kt. Seas 9 ft.\\n.THU NIGHT...E wind 15 kt. Seas 8 ft.\\n.FRI...NE wind 25 kt. Seas 9 ft.\\n.SAT...SE gale to 35 kt. Seas 12 ft.\\n.SUN...SE gale to 35 kt. Seas 15 ft.\",\n                \"instruction\": null,\n                \"response\": \"Avoid\",\n                \"parameters\": {\n                    \"AWIPSidentifier\": [\n                        \"CWFAEG\"\n                    ],\n                    \"WMOidentifier\": [\n                        \"FZAK52 PAJK 022358\"\n                    ],\n                    \"NWSheadline\": [\n                        \"SMALL CRAFT ADVISORY THROUGH WEDNESDAY\"\n                    ],\n                    \"BLOCKCHANNEL\": [\n                        \"EAS\",\n                        \"NWEM\",\n                        \"CMAS\"\n                    ],\n                    \"VTEC\": [\n                        \"/O.NEW.PAJK.SC.Y.1229.251202T2300Z-251204T0200Z/\"\n                    ],\n                    \"eventEndingTime\": [\n                        \"2025-12-03T17:00:00-09:00\"\n                    ]\n                },\n                \"scope\": \"Public\",\n                \"code\": \"IPAWSv1.0\",\n                \"language\": \"en-US\",\n                \"web\": \"http://www.weather.gov\",\n                \"eventCode\": {\n                    \"SAME\": [\n                        \"NWS\"\n                    ],\n                    \"NationalWeatherService\": [\n                        \"SCY\"\n                    ]\n                }\n            }\n        },\n        {\n            \"id\": \"https://api.weather.gov/alerts/urn:oid:2.49.0.1.840.0.63d5e98d8e0beb997c67cb867ab3ed73fdae0812.012.1\",\n            \"type\": \"Feature\",\n            \"geometry\": null,\n            \"properties\": {\n                \"@id\": \"https://api.weather.gov/alerts/urn:oid:2.49.0.1.840.0.63d5e98d8e0beb997c67cb867ab3ed73fdae0812.012.1\",\n                \"@type\": \"wx:Alert\",\n                \"id\": \"urn:oid:2.49.0.1.840.0.63d5e98d8e0beb997c67cb867ab3ed73fdae0812.012.1\",\n                \"areaDesc\": \"Icy Cape to Cape Suckling out to 15 NM\",\n                \"geocode\": {\n                    \"SAME\": [\n                        \"058652\"\n                    ],\n                    \"UGC\": [\n                        \"PKZ652\"\n                    ]\n                },\n                \"affectedZones\": [\n                    \"https://api.weather.gov/zones/forecast/PKZ652\"\n                ],\n                \"references\": [],\n                \"sent\": \"2025-12-02T14:58:00-09:00\",\n                \"effective\": \"2025-12-02T14:58:00-09:00\",\n                \"onset\": \"2025-12-02T14:00:00-09:00\",\n                \"expires\": \"2025-12-03T09:00:00-09:00\",\n                \"ends\": \"2025-12-03T17:00:00-09:00\",\n                \"status\": \"Actual\",\n                \"messageType\": \"Alert\",\n                \"category\": \"Met\",\n                \"severity\": \"Minor\",\n                \"certainty\": \"Likely\",\n                \"urgency\": \"Expected\",\n                \"event\": \"Small Craft Advisory\",\n                \"sender\": \"w-nws.webmaster@noaa.gov\",\n                \"senderName\": \"NWS Juneau AK\",\n                \"headline\": \"Small Craft Advisory issued December 2 at 2:58PM AKST until December 3 at 5:00PM AKST by NWS Juneau AK\",\n                \"description\": \"Southeast Alaska Coastal Waters from Dixon Entrance to\\nCape Suckling out 100 NM\\n\\nWind forecasts reflect the predominant speed and direction\\nexpected. Seas forecasts represent the average of the highest\\none-third of the combined windwave and swell height.\\n\\n.TONIGHT...E wind 30 kt. Seas 12 ft. Rain in the evening.\\n.WED...E wind 25 kt diminishing to 10 kt in the afternoon.\\nSeas 12 ft. Rain.\\n.WED NIGHT...W wind 10 kt. Seas 10 ft.\\n.THU...Light winds. Seas 8 ft. SW swell.\\n.THU NIGHT...E wind 10 kt. Seas 7 ft. SW swell.\\n.FRI...E wind 20 kt. Seas 7 ft.\\n.SAT...E wind 30 kt. Seas 11 ft.\\n.SUN...E gale to 35 kt. Seas 15 ft.\",\n                \"instruction\": null,\n                \"response\": \"Avoid\",\n                \"parameters\": {\n                    \"AWIPSidentifier\": [\n                        \"CWFAEG\"\n                    ],\n                    \"WMOidentifier\": [\n                        \"FZAK52 PAJK 022358\"\n                    ],\n                    \"NWSheadline\": [\n                        \"SMALL CRAFT ADVISORY THROUGH WEDNESDAY\"\n                    ],\n                    \"BLOCKCHANNEL\": [\n                        \"EAS\",\n                        \"NWEM\",\n                        \"CMAS\"\n                    ],\n                    \"VTEC\": [\n                        \"/O.NEW.PAJK.SC.Y.1233.251202T2300Z-251204T0200Z/\"\n                    ],\n                    \"eventEndingTime\": [\n                        \"2025-12-03T17:00:00-09:00\"\n                    ]\n                },\n                \"scope\": \"Public\",\n                \"code\": \"IPAWSv1.0\",\n                \"language\": \"en-US\",\n                \"web\": \"http://www.weather.gov\",\n                \"eventCode\": {\n                    \"SAME\": [\n                        \"NWS\"\n                    ],\n                    \"NationalWeatherService\": [\n                        \"SCY\"\n                    ]\n                }\n            }\n        },\n        {\n            \"id\": \"https://api.weather.gov/alerts/urn:oid:2.49.0.1.840.0.63d5e98d8e0beb997c67cb867ab3ed73fdae0812.006.1\",\n            \"type\": \"Feature\",\n            \"geometry\": null,\n            \"properties\": {\n                \"@id\": \"https://api.weather.gov/alerts/urn:oid:2.49.0.1.840.0.63d5e98d8e0beb997c67cb867ab3ed73fdae0812.006.1\",\n                \"@type\": \"wx:Alert\",\n                \"id\": \"urn:oid:2.49.0.1.840.0.63d5e98d8e0beb997c67cb867ab3ed73fdae0812.006.1\",\n                \"areaDesc\": \"Cape Edgecumbe to Cape Spencer out to 15 NM\",\n                \"geocode\": {\n                    \"SAME\": [\n                        \"058643\"\n                    ],\n                    \"UGC\": [\n                        \"PKZ643\"\n                    ]\n                },\n                \"affectedZones\": [\n                    \"https://api.weather.gov/zones/forecast/PKZ643\"\n                ],\n                \"references\": [],\n                \"sent\": \"2025-12-02T14:58:00-09:00\",\n                \"effective\": \"2025-12-02T14:58:00-09:00\",\n                \"onset\": \"2025-12-02T14:00:00-09:00\",\n                \"expires\": \"2025-12-03T09:00:00-09:00\",\n                \"ends\": \"2025-12-03T17:00:00-09:00\",\n                \"status\": \"Actual\",\n                \"messageType\": \"Alert\",\n                \"category\": \"Met\",\n                \"severity\": \"Minor\",\n                \"certainty\": \"Likely\",\n                \"urgency\": \"Expected\",\n                \"event\": \"Small Craft Advisory\",\n                \"sender\": \"w-nws.webmaster@noaa.gov\",\n                \"senderName\": \"NWS Juneau AK\",\n                \"headline\": \"Small Craft Advisory issued December 2 at 2:58PM AKST until December 3 at 5:00PM AKST by NWS Juneau AK\",\n                \"description\": \"Southeast Alaska Coastal Waters from Dixon Entrance to\\nCape Suckling out 100 NM\\n\\nWind forecasts reflect the predominant speed and direction\\nexpected. Seas forecasts represent the average of the highest\\none-third of the combined windwave and swell height.\\n\\n.TONIGHT...SE wind 20 kt. Seas 11 ft. Rain.\\n.WED...SE wind 20 kt becoming SW in the afternoon. Seas\\n11 ft. SW swell. Rain in the morning.\\n.WED NIGHT...W wind 20 kt. Seas 10 ft.\\n.THU...W wind 10 kt. Seas 9 ft.\\n.THU NIGHT...E wind 15 kt. Seas 8 ft.\\n.FRI...NE wind 20 kt. Seas 10 ft.\\n.SAT...S wind 30 kt. Seas 12 ft.\\n.SUN...S wind 30 kt. Seas 16 ft.\",\n                \"instruction\": null,\n                \"response\": \"Avoid\",\n                \"parameters\": {\n                    \"AWIPSidentifier\": [\n                        \"CWFAEG\"\n                    ],\n                    \"WMOidentifier\": [\n                        \"FZAK52 PAJK 022358\"\n                    ],\n                    \"NWSheadline\": [\n                        \"SMALL CRAFT ADVISORY THROUGH WEDNESDAY\"\n                    ],\n                    \"BLOCKCHANNEL\": [\n                        \"EAS\",\n                        \"NWEM\",\n                        \"CMAS\"\n                    ],\n                    \"VTEC\": [\n                        \"/O.NEW.PAJK.SC.Y.1227.251202T2300Z-251204T0200Z/\"\n                    ],\n                    \"eventEndingTime\": [\n                        \"2025-12-03T17:00:00-09:00\"\n                    ]\n                },\n                \"scope\": \"Public\",\n                \"code\": \"IPAWSv1.0\",\n                \"language\": \"en-US\",\n                \"web\": \"http://www.weather.gov\",\n                \"eventCode\": {\n                    \"SAME\": [\n                        \"NWS\"\n                    ],\n                    \"NationalWeatherService\": [\n                        \"SCY\"\n                    ]\n                }\n            }\n        },\n        {\n            \"id\": \"https://api.weather.gov/alerts/urn:oid:2.49.0.1.840.0.63d5e98d8e0beb997c67cb867ab3ed73fdae0812.007.1\",\n            \"type\": \"Feature\",\n            \"geometry\": null,\n            \"properties\": {\n                \"@id\": \"https://api.weather.gov/alerts/urn:oid:2.49.0.1.840.0.63d5e98d8e0beb997c67cb867ab3ed73fdae0812.007.1\",\n                \"@type\": \"wx:Alert\",\n                \"id\": \"urn:oid:2.49.0.1.840.0.63d5e98d8e0beb997c67cb867ab3ed73fdae0812.007.1\",\n                \"areaDesc\": \"Cape Edgecumbe to Cape Spencer from 15 to 80 NM\",\n                \"geocode\": {\n                    \"SAME\": [\n                        \"058663\"\n                    ],\n                    \"UGC\": [\n                        \"PKZ663\"\n                    ]\n                },\n                \"affectedZones\": [\n                    \"https://api.weather.gov/zones/forecast/PKZ663\"\n                ],\n                \"references\": [],\n                \"sent\": \"2025-12-02T14:58:00-09:00\",\n                \"effective\": \"2025-12-02T14:58:00-09:00\",\n                \"onset\": \"2025-12-02T14:00:00-09:00\",\n                \"expires\": \"2025-12-03T09:00:00-09:00\",\n                \"ends\": \"2025-12-03T17:00:00-09:00\",\n                \"status\": \"Actual\",\n                \"messageType\": \"Alert\",\n                \"category\": \"Met\",\n                \"severity\": \"Minor\",\n                \"certainty\": \"Likely\",\n                \"urgency\": \"Expected\",\n                \"event\": \"Small Craft Advisory\",\n                \"sender\": \"w-nws.webmaster@noaa.gov\",\n                \"senderName\": \"NWS Juneau AK\",\n                \"headline\": \"Small Craft Advisory issued December 2 at 2:58PM AKST until December 3 at 5:00PM AKST by NWS Juneau AK\",\n                \"description\": \"Southeast Alaska Coastal Waters from Dixon Entrance to\\nCape Suckling out 100 NM\\n\\nWind forecasts reflect the predominant speed and direction\\nexpected. Seas forecasts represent the average of the highest\\none-third of the combined windwave and swell height.\\n\\n.TONIGHT...S wind 20 kt. Seas 12 ft. Rain in the evening.\\n.WED...S wind 15 kt becoming W in the afternoon. Seas\\n11 ft. SW swell.\\n.WED NIGHT...W wind 20 kt. Seas 10 ft.\\n.THU...W wind 15 kt. Seas 9 ft.\\n.THU NIGHT...SE wind 20 kt. Seas 9 ft.\\n.FRI...SW wind 20 kt. Seas 10 ft.\\n.SAT...S wind 30 kt. Seas 14 ft.\\n.SUN...S wind 30 kt. Seas 19 ft.\",\n                \"instruction\": null,\n                \"response\": \"Avoid\",\n                \"parameters\": {\n                    \"AWIPSidentifier\": [\n                        \"CWFAEG\"\n                    ],\n                    \"WMOidentifier\": [\n                        \"FZAK52 PAJK 022358\"\n                    ],\n                    \"NWSheadline\": [\n                        \"SMALL CRAFT ADVISORY THROUGH WEDNESDAY\"\n                    ],\n                    \"BLOCKCHANNEL\": [\n                        \"EAS\",\n                        \"NWEM\",\n                        \"CMAS\"\n                    ],\n                    \"VTEC\": [\n                        \"/O.NEW.PAJK.SC.Y.1228.251202T2300Z-251204T0200Z/\"\n                    ],\n                    \"eventEndingTime\": [\n                        \"2025-12-03T17:00:00-09:00\"\n                    ]\n                },\n                \"scope\": \"Public\",\n                \"code\": \"IPAWSv1.0\",\n                \"language\": \"en-US\",\n                \"web\": \"http://www.weather.gov\",\n                \"eventCode\": {\n                    \"SAME\": [\n                        \"NWS\"\n                    ],\n                    \"NationalWeatherService\": [\n                        \"SCY\"\n                    ]\n                }\n            }\n        },\n        {\n            \"id\": \"https://api.weather.gov/alerts/urn:oid:2.49.0.1.840.0.63d5e98d8e0beb997c67cb867ab3ed73fdae0812.010.1\",\n            \"type\": \"Feature\",\n            \"geometry\": null,\n            \"properties\": {\n                \"@id\": \"https://api.weather.gov/alerts/urn:oid:2.49.0.1.840.0.63d5e98d8e0beb997c67cb867ab3ed73fdae0812.010.1\",\n                \"@type\": \"wx:Alert\",\n                \"id\": \"urn:oid:2.49.0.1.840.0.63d5e98d8e0beb997c67cb867ab3ed73fdae0812.010.1\",\n                \"areaDesc\": \"Cape Fairweather to Icy Cape out to 15 NM\",\n                \"geocode\": {\n                    \"SAME\": [\n                        \"058651\"\n                    ],\n                    \"UGC\": [\n                        \"PKZ651\"\n                    ]\n                },\n                \"affectedZones\": [\n                    \"https://api.weather.gov/zones/forecast/PKZ651\"\n                ],\n                \"references\": [],\n                \"sent\": \"2025-12-02T14:58:00-09:00\",\n                \"effective\": \"2025-12-02T14:58:00-09:00\",\n                \"onset\": \"2025-12-02T14:00:00-09:00\",\n                \"expires\": \"2025-12-03T09:00:00-09:00\",\n                \"ends\": \"2025-12-03T17:00:00-09:00\",\n                \"status\": \"Actual\",\n                \"messageType\": \"Alert\",\n                \"category\": \"Met\",\n                \"severity\": \"Minor\",\n                \"certainty\": \"Likely\",\n                \"urgency\": \"Expected\",\n                \"event\": \"Small Craft Advisory\",\n                \"sender\": \"w-nws.webmaster@noaa.gov\",\n                \"senderName\": \"NWS Juneau AK\",\n                \"headline\": \"Small Craft Advisory issued December 2 at 2:58PM AKST until December 3 at 5:00PM AKST by NWS Juneau AK\",\n                \"description\": \"Southeast Alaska Coastal Waters from Dixon Entrance to\\nCape Suckling out 100 NM\\n\\nWind forecasts reflect the predominant speed and direction\\nexpected. Seas forecasts represent the average of the highest\\none-third of the combined windwave and swell height.\\n\\n.TONIGHT...E wind 20 kt. Seas 10 ft. Rain.\\n.WED...SE wind 25 kt becoming SW 15 kt in the afternoon.\\nSeas 12 ft. Rain.\\n.WED NIGHT...W wind 15 kt. Seas 10 ft.\\n.THU...W wind 10 kt. Seas 8 ft. SW swell.\\n.THU NIGHT...E wind 10 kt. Seas 7 ft. SW swell.\\n.FRI...E wind 25 kt. Seas 9 ft.\\n.SAT...E gale to 35 kt. Seas 12 ft.\\n.SUN...E gale to 35 kt. Seas 15 ft.\",\n                \"instruction\": null,\n                \"response\": \"Avoid\",\n                \"parameters\": {\n                    \"AWIPSidentifier\": [\n                        \"CWFAEG\"\n                    ],\n                    \"WMOidentifier\": [\n                        \"FZAK52 PAJK 022358\"\n                    ],\n                    \"NWSheadline\": [\n                        \"SMALL CRAFT ADVISORY THROUGH WEDNESDAY\"\n                    ],\n                    \"BLOCKCHANNEL\": [\n                        \"EAS\",\n                        \"NWEM\",\n                        \"CMAS\"\n                    ],\n                    \"VTEC\": [\n                        \"/O.NEW.PAJK.SC.Y.1231.251202T2300Z-251204T0200Z/\"\n                    ],\n                    \"eventEndingTime\": [\n                        \"2025-12-03T17:00:00-09:00\"\n                    ]\n                },\n                \"scope\": \"Public\",\n                \"code\": \"IPAWSv1.0\",\n                \"language\": \"en-US\",\n                \"web\": \"http://www.weather.gov\",\n                \"eventCode\": {\n                    \"SAME\": [\n                        \"NWS\"\n                    ],\n                    \"NationalWeatherService\": [\n                        \"SCY\"\n                    ]\n                }\n            }\n        },\n        {\n            \"id\": \"https://api.weather.gov/alerts/urn:oid:2.49.0.1.840.0.63d5e98d8e0beb997c67cb867ab3ed73fdae0812.005.1\",\n            \"type\": \"Feature\",\n            \"geometry\": null,\n            \"properties\": {\n                \"@id\": \"https://api.weather.gov/alerts/urn:oid:2.49.0.1.840.0.63d5e98d8e0beb997c67cb867ab3ed73fdae0812.005.1\",\n                \"@type\": \"wx:Alert\",\n                \"id\": \"urn:oid:2.49.0.1.840.0.63d5e98d8e0beb997c67cb867ab3ed73fdae0812.005.1\",\n                \"areaDesc\": \"Cape Decision to Cape Edgecumbe from 15 to 80 NM\",\n                \"geocode\": {\n                    \"SAME\": [\n                        \"058662\"\n                    ],\n                
